vi "sendValue.vi"(8 "error in (no error)":errorcluster, 10 "data":variant, 11 "allAxisInPosition in":refnum<class "allAxisInPosition.lvclass">) -> (0 "error out":errorcluster, 2 "function return":i32, 3 "allAxisInPosition out":refnum<class "allAxisInPosition.lvclass">)   [LabVIEW 2016, in "SALLV_AtDome_Messaging.lvlib" / "allAxisInPosition.lvclass"]
uses:
  allAxisInPosition.lvclass
  ts_sallv_AtDome/DataTypes/logevent_allAxisInPosition.ctl
  ts_sallv_AtDome/SALLV_AtDome.lvlib
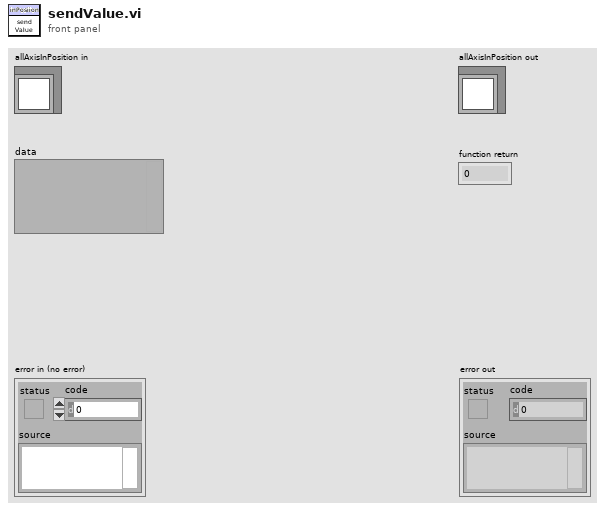
[diagram p1: front panel]
types:
  T1 = typedef "SALLV_AtDome.lvlib/logevent_allAxisInPosition.ctl" = cluster{"inPosition":bool, "priority":i32}
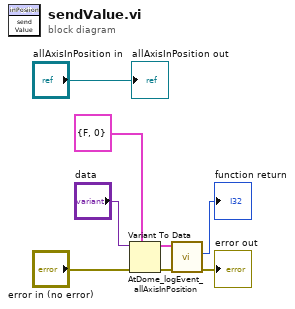
[diagram p0: block diagram]
diagram:
  n1 = Variant To Data(error in="error in (no error)", type=T1 {"inPosition"=FALSE, "priority"=0} ("logevent_allAxisInPosition_Ctl"), Variant="data") -> (data=w4:T1, error out=w5:errorcluster)
  n2 = call "AtDome_logEvent_allAxisInPosition.vi"("error in (no error)"=w5, "logevent_allAxisInPosition_Ctl"=w4) -> ("error out"=→"error out":errorcluster, "function return"=→"function return":i32)  [unwired: 7 in, 1 out]
  "allAxisInPosition out" <- "allAxisInPosition in"
